vi "Open Device.vi"(0 "fpga ref":refnum<k20>, 11 "error in":errorcluster) -> (4 "Register Bus (out)":T1, 15 "error out":errorcluster)   [LabVIEW 2017]
doc: "Opens a session to the NI-579x Configuration Design Library. Creates a session to the Register Bus Host library and initializes the CLIP.\n\n<B>Input Parameters</B>\n\n<B>fpga ref</B> is a reference to a LabVIEW FPGA created using the Open FPGA VI Reference VI.\n\n<B>error in</B> describes error conditions that occur before this node runs. This input provides standard 'error in' functionality.\n\n<B>Output Parameters</B>\n\n<B>Register Bus (out)</B> is a new Register Bus session used in all subsequent NI-579x Configuration Design Library Host VIs.\n\n<B>error out</B> contains error information. This output provides standard 'error out' functionality."
uses:
  <instrlib>/_niInstr/Register Bus/v0/Host/Public/Register Bus Session.ctl
  <instrlib>/_niInstr/Register Bus/v0/Host/Private/Session Data.ctl
  <instrlib>/ni579x/Config/v2/Host/ni579x Config v2 Host.lvlib
  <instrlib>/_niInstr/Register Bus/v0/Host/niInstr Register Bus v0 Host.lvlib
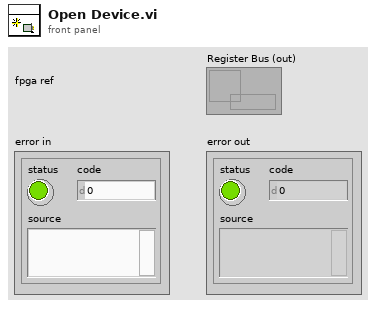
[diagram p1: front panel]
types:
  T1 = typedef "niInstr Register Bus v0 Host.lvlib/Register Bus Session.ctl" = refnum<queue>
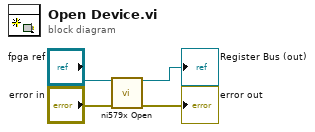
[diagram p0: block diagram]
diagram:
  n1 = call <instrlib>:"ni579x Open.vi"("fpga ref"="fpga ref", "Error In"="error in") -> ("Register Bus (out)"=→"Register Bus (out)":T1, "Error Out"=→"error out":errorcluster)  [unwired: 12 in]
